vi "Web_Client_low.vi"(0 "Channel Name":string="Froude:NPL:Atmos_Press", 1 "Extra Info":string) -> (2 "Header String":string, 3 "Data Read":string, 4 "Comms Error":bool, 5 "Number of lines read":i32)   [LabVIEW 2010]
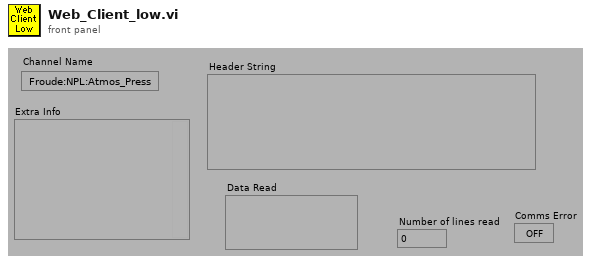
[diagram p1: front panel]
types:
  T1 = enum16{"Standard", "Buffered", "CRLF", "Immediate"}
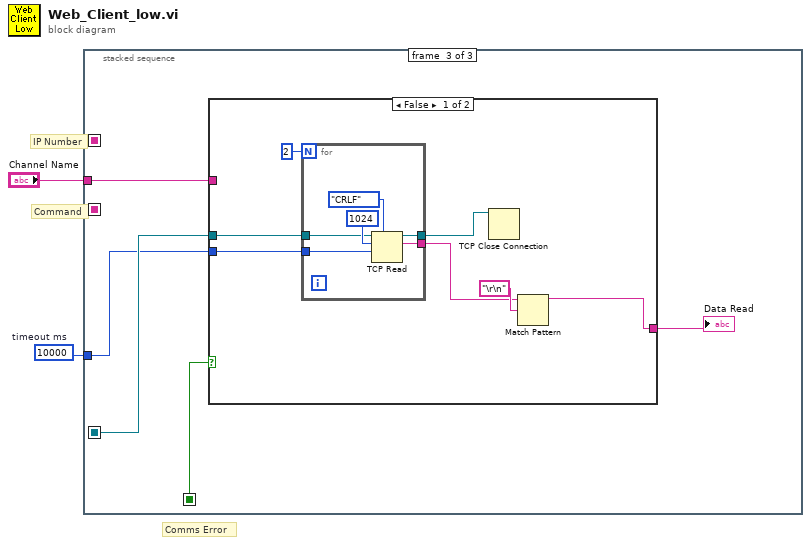
[diagram p0: block diagram]
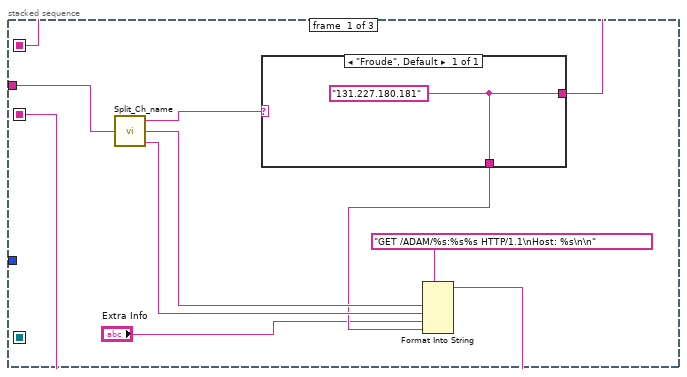
[diagram p2: hidden frame]
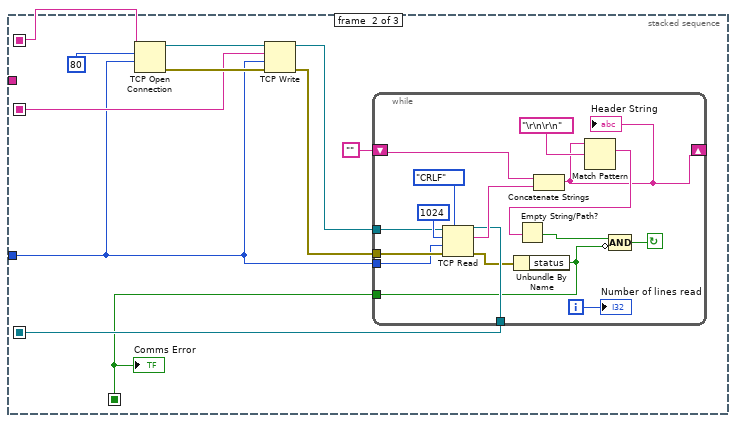
[diagram p3: hidden frame]
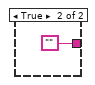
[diagram p4: hidden frame]
diagram:
  w1 = 10000  # timeout ms
  # "Comms Error"
  # "Command"
  # "IP Number"
  n1 = stacked-sequence {
    seq-local: [_ w18 _] -> [_ _ w44]
    seq-local: [w7 _ _] -> [_ w16 _]
    seq-local: [w6 _ _] -> [_ w17 _]
    seq-local: [_ w13 _] -> [_ _ w43]
    tunnel: "Channel Name" -> [w5 _ w42]
    tunnel: w1 -> [_ w14 w41]
    frame #0 {
      n2 = call "Split_Ch_name.vi"("Ch name"=w5) -> ("Top level"=w11:string, "Middle"=w9:string, "Low level"=w8:string)
      n3 = case shown="\"Froude\", Default" w11 {
        tunnel: [w12] -> w7
        tunnel: [w12] -> w4
        frame "Froude", Default {
          w12 = "131.227.180.181" ("Hostname")
        }
      }
      n4 = Format Into String(format string="GET /ADAM/%s:%s%s HTTP/1.1\nHost: %s\n\n" ("data in"), w9, w8, "Extra Info", w4) -> (resulting string=w6:string)  [unwired: 2 in, 1 out]
    }
    frame #1 {
      n5 = TCP Open Connection(address=w16, remote port or service name=u16 80, timeout ms (60000)=w14) -> (connection ID=w22:refnum<k5>, error out=w21:errorcluster)  [unwired: 2 in]
      n6 = TCP Write(connection ID=w22, data in=w17, error in (no error)=w21, 9:w14) -> (connection ID out=w20:refnum<k5>, error out=w15:errorcluster)  [unwired: 1 out]
      n7 = while {
        tunnel: [w24] -> w13
        tunnel: w14 -> [w28]
        tunnel: w15 -> [w29]
        tunnel: [w30] -> w18
        shift-left: "" -> [w35]
        shift-right: [w32] -> _
        tunnel: w20 -> [w31]
        i -> [w37]
        stop <- w25 continue-if-true
        n8 = TCP Read(connection ID=w31, bytes to read=1024, error in (no error)=w29, 7:T1."CRLF" ("mode (standard)"), 9:w28) -> (connection ID out=w30:refnum<k5>, data out=w34:string, error out=w27:errorcluster)
        n9 = Unbundle By Name(w27) -> ("status"=w24:bool)
        n10 = Concatenate Strings(w35, w34) -> (w32:string)
        "Header String" <- w32
        n11 = Match Pattern(string=w32, regular expression="\r\n\r\n") -> (match substring=w33:string)  [unwired: 1 in, 3 out]
        n12 = Empty String/Path?(string/path=w33) -> (empty?=w26:bool)
        n13 = Compound Arithmetic op=AND(w26, invert w24) -> (w25:bool)
        "Number of lines read" <- w37
      }
      "Comms Error" <- w13
    }
    frame #2 {
      n14 = case shown="False" w43 {
        tunnel: w44 -> [w49 _]
        tunnel: w42 -> [_ _]
        tunnel: w41 -> [w48 _]
        tunnel: [w45 ""] -> w40
        frame False {
          n15 = for {
            N: 2 -> [_]
            tunnel: w49 -> [w55]
            tunnel: [w53] -> w46
            tunnel: [w54] -> w50
            tunnel: w48 -> [w52]
            n16 = TCP Read(connection ID=w55, bytes to read=1024, 7:T1."CRLF" ("mode (standard)"), 9:w52) -> (connection ID out=w54:refnum<k5>, data out=w53:string)  [unwired: 1 in, 1 out]
          }
          n17 = TCP Close Connection(connection ID=w50) -> ()  [unwired: 2 in, 2 out]
          n18 = Match Pattern(string=w46, regular expression="\r\n" ("String to match")) -> (before substring=w45:string)  [unwired: 1 in, 3 out]
        }
        frame True {
        }
      }
      "Data Read" <- w40
    }
  }
